vi "Replace AO and REF Ch.vi"(8 "error in (no error)":errorcluster, 10 "Instrument.DAQ (NEW)":refnum<class "Instrument.DAQ.lvclass">, 11 "Instrument.DAQ (OLD)":refnum<class "Instrument.DAQ.lvclass">) -> (0 "error out":errorcluster, 3 "Instrument.DAQ out":refnum<class "Instrument.DAQ.lvclass">)   [LabVIEW 2019, in "Instrument.Lockin.lvlib" / "Instrument.DAQ.lvclass"]
uses:
  Instrument.DAQ.lvclass
  Instrument.DAQ.lvclass/Instrument.DAQ.ctl
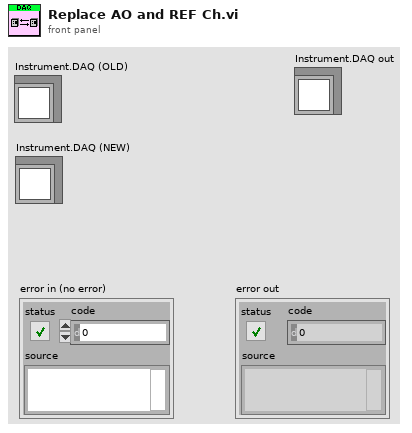
[diagram p1: front panel]
types:
  T1 = typedef "Instrument.Lockin.lvlib/Instrument.DAQ.lvclass/AO.Channel--Cluster--Array.ctl" = T2[]
  T2 = typedef "Instrument.Lockin.lvlib/Instrument.DAQ.lvclass/AO.Channel--Cluster.ctl" = cluster{"Enable?":bool, "Channel":i32, "Amplitude":dbl, "Offset":dbl, "Frequency":dbl, "Phase":dbl, "Function":T3, "Sweeping?":bool, "Limit AC":bool, "Limit DC?":bool, "Duty Cycle":bool}
  T3 = typedef "Instrument.Lockin.lvlib/Instrument.DAQ.lvclass/AO.Channel.Function--Enum.ctl" = enum16{"sine", "square", "triangle", "saw"}
  T4 = typedef "Instrument.Lockin.lvlib/Instrument.DAQ.lvclass/REF.Channel--Cluster--Array.ctl" = T5[]
  T5 = typedef "Instrument.Lockin.lvlib/Instrument.DAQ.lvclass/REF.Channel--Cluster.ctl" = cluster{"Enable?":bool, "Channel":i32, "Frequency":dbl, "Phase":dbl, "TC":dbl, "Roll-Off":i32}
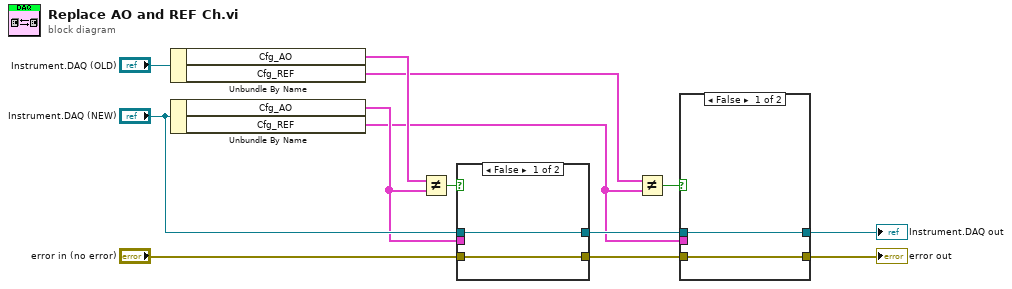
[diagram p0: block diagram]
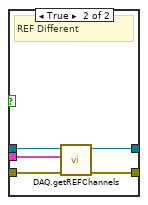
[diagram p2: hidden frame]
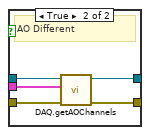
[diagram p3: hidden frame]
diagram:
  n1 = Unbundle By Name("Instrument.DAQ (OLD)") -> ("Cfg_AO"=w4:T1, "Cfg_REF"=w2:T4)
  n2 = Unbundle By Name("Instrument.DAQ (NEW)") -> ("Cfg_AO"=w3:T1, "Cfg_REF"=w1:T4)
  n3 = Not Equal?(x=w4, y=w3) -> (x != y?=w12:bool)
  n4 = case shown="False" w12 {
    tunnel: [w15 w19] -> w9
    tunnel: "Instrument.DAQ (NEW)" -> [w15 w20]
    tunnel: "error in (no error)" -> [w14 w18]
    tunnel: [w14 w17] -> w7
    tunnel: w3 -> [_ w16]
    frame False {
    }
    frame True {
      # "AO Different"
      n5 = call "DAQ.getAOChannels.vi"("error in (no error)"=w18, "Channels: AO"=w16, "Instrument.DAQ"=w20) -> ("error out"=w17:errorcluster, "Instrument.DAQ out"=w19:refnum<class "Instrument.DAQ.lvclass">)  [unwired: 7 in]
    }
  }
  n6 = Not Equal?(x=w2, y=w1) -> (x != y?=w11:bool)
  n7 = case shown="False" w11 {
    tunnel: [w22 w26] -> w10
    tunnel: w9 -> [w22 w27]
    tunnel: w7 -> [w21 w25]
    tunnel: [w21 w24] -> w6
    tunnel: w1 -> [_ w23]
    frame False {
    }
    frame True {
      # "REF Different"
      n8 = call "DAQ.getREFChannels.vi"("error in (no error)"=w25, "Channels.REF"=w23, "Instrument.DAQ"=w27) -> ("error out"=w24:errorcluster, "Instrument.DAQ out"=w26:refnum<class "Instrument.DAQ.lvclass">)  [unwired: 7 in]
    }
  }
  "Instrument.DAQ out" <- w10
  "error out" <- w6
